vi "mem mgr tester.vi"   [LabVIEW 2015]
uses:
  <vilib>/rvi/Emulation/niFpgaGetClockAttributes.vi
  <vilib>/rvi/Emulation/niFpgaSctlEmulationGetInTimedLoop.vi
  <vilib>/rvi/Emulation/niFpgaEmulationReportErrorSimple.vi
  <vilib>/rvi/Emulation/niFpgaEmulationIsFPGAContextNoSignature.vi
  <vilib>/rvi/errors/niFpgaSetErrorForExecOnDevCompSimple.vi
  <vilib>/rvi/eio/common/nirviEmuReportErrorAndStop.vi
  <vilib>/rvi/DataTransferAndStorage/Container/Common/niFpgaContainerGetUniqueNameForEmu.vi
  <vilib>/rvi/FIFO/Fifo_Resource/nirvififoEmulationSetSize.vi
  <vilib>/rvi/FIFO/Fifo_Resource/nirviFifoEmulationQueueMgr.vi
  <instcachedir>/0/nirviFifoEmulationQueueMgr_E5CAEC123FF24DC58D834DCA3CDAA9B5.lvgen/nirviFifoEmulationQueueMgr_E5CAEC123FF24DC58D834DCA3CDAA9B5_000.vi
  <vilib>/rvi/FIFO/Fifo_Resource/nirvififoEmulationDetermineInputValidOut.vi
  <vilib>/rvi/FIFO/Fifo_Resource/nirvififoEmulationCreateLock.vi
  <vilib>/rvi/Emulation/niFpgaProcessEmulError.vi
  <vilib>/rvi/FIFO/Fifo_Resource/nirvififoEmulationObtainLock.vi
  <vilib>/rvi/FIFO/Fifo_Resource/nirvififoEmulationReleaseLock.vi
  <vilib>/rvi/occurrence/nirviWaitOnOccurrenceBase.vi
  <vilib>/rvi/errors/nirviReportUnexpectedCaseInternalError.vi
  <vilib>/rvi/errors/nirviReportUnexpectedCaseInternalError (U32).vi
  <vilib>/rvi/Emulation/niFpgaCriticalErrorInLSC.vi
  <vilib>/Utility/error.llb/Clear Errors.vi
  <vilib>/rvi/DataTransferAndStorage/Container/XNode/niFpgaContainer.xnode
  <vilib>/rvi/FIFO/Fifo_Resource/nirvififoEmulationWrite.vi
  <vilib>/rvi/FIFO/Fifo_Resource/nirvififoEmulationRead.vi
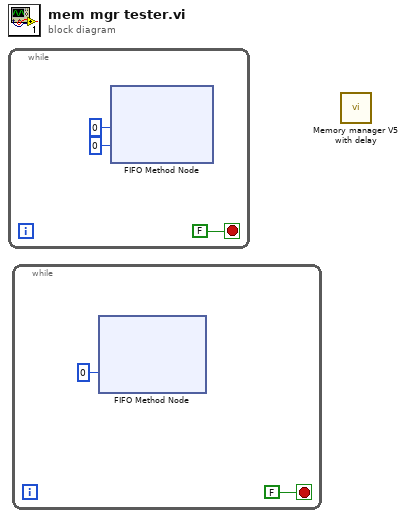
[diagram p0: block diagram]
diagram:
  n1 = while {
    stop <- FALSE stop-if-true
    n2 = xnode ("FIFO Method Node")("Element"=u32 0, "Timeout"=0) -> ()  [unwired: 1 in, 2 out]
  }
  n3 = while {
    stop <- FALSE stop-if-true
    n4 = xnode ("FIFO Method Node")("Timeout"=0) -> ()  [unwired: 1 in, 3 out]
  }
  n5 = call "Memory manager V5 with delay.vi"() -> ()  [unwired: 12 in]
